vi "Read Image Pixel Data FIFO.vi"(0 "fpga inteface in":refnum<k20>, 5 "display channel number":i32, 7 "number of elements":u32, 11 "error in (no error)":errorcluster) -> (4 "fpga interface out":refnum<k20>, 6 "image pixel data region":refnum<data-value>, 8 "elements in region":u32, 10 "elements remaining":u32, 15 "error out":errorcluster)   [LabVIEW 2025, in "GettingStarted_Common_148X_Host.lvlib"]
uses:
  GettingStarted_Common_148X_Host.lvlib
  Types/148x_Common_FPGA_Reference.ctl
  <vilib>/rvi/errors/niLvFpgaAdjustHostInterfaceError.vi
  <vilib>/rvi/interface/nirviMethod/nirviMethod.xnode
  <vilib>/rvi/errors/niLvFpgaMergeErrorWithErrorCode.vi
  <vilib>/FPGAPlugInAG/Dynamic/niLvFpga_AcquireReadRegionFifo_Dynamic.vi
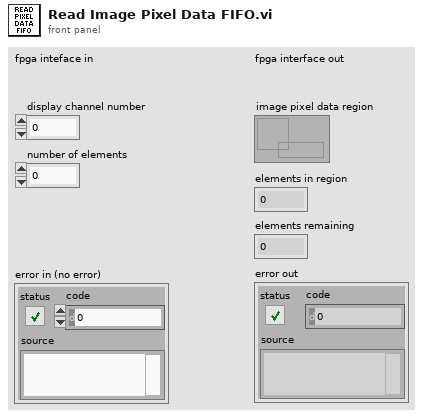
[diagram p1: front panel]
types:
  T1 = typedef "GettingStarted_Common_148X_Host.lvlib/148x_Common_FPGA_Reference.ctl" = refnum<k20>
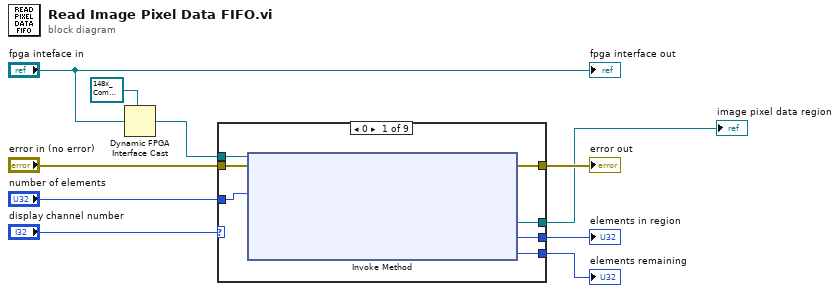
[diagram p0: block diagram]
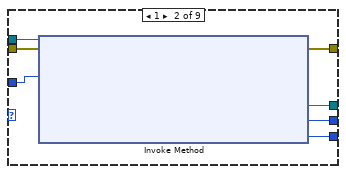
[diagram p2: hidden frame]
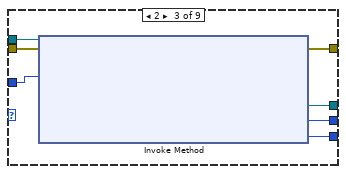
[diagram p3: hidden frame]
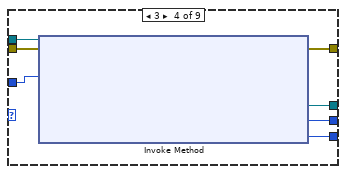
[diagram p4: hidden frame]
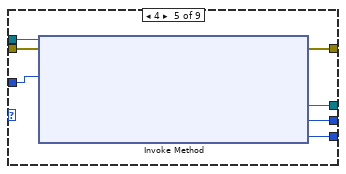
[diagram p5: hidden frame]
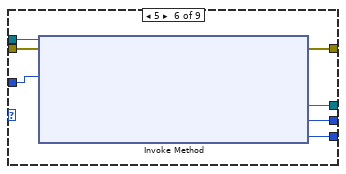
[diagram p6: hidden frame]
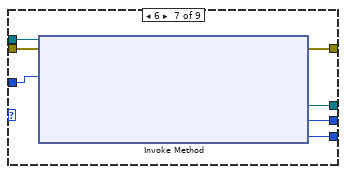
[diagram p7: hidden frame]
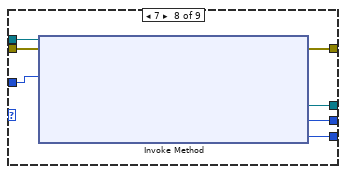
[diagram p8: hidden frame]
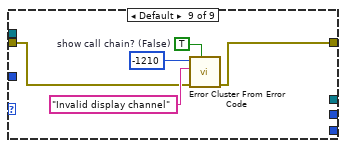
[diagram p9: hidden frame]
diagram:
  n1 = Dynamic FPGA Interface Cast(Session In=T1 refnum ("FPGA VI Reference Out"), Type="fpga inteface in") -> (Session Out=w8:T1)
  n2 = case shown="0" "display channel number" {
    tunnel: "error in (no error)" -> [w17 w24 w31 w38 w45 w52 w59 w66 w68]
    tunnel: w8 -> [w16 w23 w30 w37 w44 w51 w58 w65 _]
    tunnel: [w15 w22 w29 w36 w43 w50 w57 w64 w67] -> w4
    tunnel: "number of elements" -> [w14 w21 w28 w35 w42 w49 w56 w63 _]
    tunnel: [w13 w20 w27 w34 w41 w48 w55 w62 _] -> w1
    tunnel: [w12 w19 w26 w33 w40 w47 w54 w61 _] -> w2
    tunnel: [w11 w18 w25 w32 w39 w46 w53 w60 _] -> w3
    frame 0 {
      n3 = xnode "Invoke Method"("FPGA VI Reference In"=w16, "error in"=w17, "Number of Elements"=w14) -> ("error out"=w15:errorcluster, "Read Region Reference"=w13:refnum<data-value>, "Elements In Region"=w12:u32, "Elements Remaining"=w11:u32)  [unwired: 1 in, 1 out]
    }
    frame 1 {
      n4 = xnode "Invoke Method"("FPGA VI Reference In"=w23, "error in"=w24, "Number of Elements"=w21) -> ("error out"=w22:errorcluster, "Read Region Reference"=w20:refnum<data-value>, "Elements In Region"=w19:u32, "Elements Remaining"=w18:u32)  [unwired: 1 in, 1 out]
    }
    frame 2 {
      n5 = xnode "Invoke Method"("FPGA VI Reference In"=w30, "error in"=w31, "Number of Elements"=w28) -> ("error out"=w29:errorcluster, "Read Region Reference"=w27:refnum<data-value>, "Elements In Region"=w26:u32, "Elements Remaining"=w25:u32)  [unwired: 1 in, 1 out]
    }
    frame 3 {
      n6 = xnode "Invoke Method"("FPGA VI Reference In"=w37, "error in"=w38, "Number of Elements"=w35) -> ("error out"=w36:errorcluster, "Read Region Reference"=w34:refnum<data-value>, "Elements In Region"=w33:u32, "Elements Remaining"=w32:u32)  [unwired: 1 in, 1 out]
    }
    frame 4 {
      n7 = xnode "Invoke Method"("FPGA VI Reference In"=w44, "error in"=w45, "Number of Elements"=w42) -> ("error out"=w43:errorcluster, "Read Region Reference"=w41:refnum<data-value>, "Elements In Region"=w40:u32, "Elements Remaining"=w39:u32)  [unwired: 1 in, 1 out]
    }
    frame 5 {
      n8 = xnode "Invoke Method"("FPGA VI Reference In"=w51, "error in"=w52, "Number of Elements"=w49) -> ("error out"=w50:errorcluster, "Read Region Reference"=w48:refnum<data-value>, "Elements In Region"=w47:u32, "Elements Remaining"=w46:u32)  [unwired: 1 in, 1 out]
    }
    frame 6 {
      n9 = xnode "Invoke Method"("FPGA VI Reference In"=w58, "error in"=w59, "Number of Elements"=w56) -> ("error out"=w57:errorcluster, "Read Region Reference"=w55:refnum<data-value>, "Elements In Region"=w54:u32, "Elements Remaining"=w53:u32)  [unwired: 1 in, 1 out]
    }
    frame 7 {
      n10 = xnode "Invoke Method"("FPGA VI Reference In"=w65, "error in"=w66, "Number of Elements"=w63) -> ("error out"=w64:errorcluster, "Read Region Reference"=w62:refnum<data-value>, "Elements In Region"=w61:u32, "Elements Remaining"=w60:u32)  [unwired: 1 in, 1 out]
    }
    frame Default {
      w69 = TRUE  # show call chain? (False)
      n11 = call <vilib>:"Error Cluster From Error Code.vi"("show call chain? (False)"=w69, "error in (no error)"=w68, "error message (\"\")"="Invalid display channel" ("error message (\"\")"), "error code (0)"=-1210) -> ("error out"=w67:errorcluster)  [unwired: 5 in]
    }
  }
  "elements remaining" <- w3
  "error out" <- w4
  "image pixel data region" <- w1
  "elements in region" <- w2
  "fpga interface out" <- "fpga inteface in"
